vi "getSerializedData.vi"(0 "reference":refnum<class "PackageNode.lvclass">, 5 "error in (no error)":errorcluster) -> (14 "reference out":refnum<class "PackageNode.lvclass">, 15 "parent":refnum<class "AbstractNode.lvclass">, 16 "children":refnum<class "AbstractNode.lvclass">[](array[class]), 17 "xmlOut":string, 19 "error out":errorcluster)   [LabVIEW 2014, in "PackageNode.lvclass"]
doc: "getSerializedData"
uses:
  <resource>/Framework/Providers/Open_GDS/UML/PackageNode_class/PackageNode.lvclass
  <resource>/Framework/Providers/Open_GDS/UML/AbstractNode_class/AbstractNode.lvclass
  <resource>/Framework/Providers/Open_GDS/UML/AbstractNode_class/ObjectReference.ctl
  <resource>/Framework/Providers/Open_GDS/UML/General/Rectangle/Rectangle Rectangle2D.ctl
  <resource>/Framework/Providers/Open_GDS/UML/MultiLineString_class/ObjectReference.ctl
  <resource>/Framework/Providers/Open_GDS/UML/MultiLineString_class/MultiLineString.lvclass
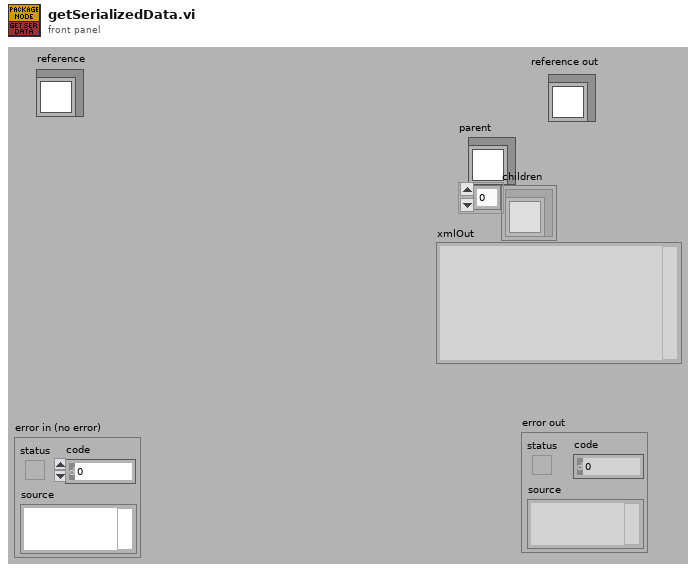
[diagram p1: front panel]
types:
  T1 = typedef "AbstractNode.lvclass/ObjectReference.ctl" = refnum<k1>
  T2 = typedef "Rectangle Rectangle2D.ctl" = cluster{"x":dbl, "y":dbl, "width":dbl, "height":dbl}
  T3 = typedef "MultiLineString.lvclass/ObjectReference.ctl" = refnum<k1>
  T4 = cluster{"Base class":cluster{"Base class":cluster{"parent":T1, "children":T1[], "Hidden":bool}, "bounds":T2}, "name":string, "contents":T3, "DEFAULT_TOP_WIDTH":i32, "DEFAULT_TOP_HEIGHT":i32, "DEFAULT_WIDTH":i32, "DEFAULT_HEIGHT":i32, "NAME_GAP":i32, "XGAP":i32, "YGAP":i32, "Collapsed":bool, "Note color":u32, "Justification":u16}
  T5 = typedef "PackageNode.lvclass/ObjectAttributes.ctl" = cluster{"Base class":T6, "name":string, "contents":refnum<class "MultiLineString.lvclass">, "DEFAULT_TOP_WIDTH":i32, "DEFAULT_TOP_HEIGHT":i32, "DEFAULT_WIDTH":i32, "DEFAULT_HEIGHT":i32, "NAME_GAP":i32, "XGAP":i32, "YGAP":i32, "Collapsed":bool, "Note color":u32, "Justification":u16}
  T6 = typedef "RectangularNode.lvclass/ObjectAttributes.ctl" = cluster{"Base class":T7, "bounds":T2}
  T7 = typedef "AbstractNode.lvclass/ObjectAttributes.ctl" = cluster{"parent":refnum<class "AbstractNode.lvclass">, "children":refnum<class "AbstractNode.lvclass">[], "Hidden":bool}
  T8 = cluster{"Attributes":cluster{"Base class":cluster{"Base class":cluster{"parent":T1, "children":T1[], "Hidden":bool}, "bounds":T2}, "name":string, "contents":T3, "DEFAULT_TOP_WIDTH":i32, "DEFAULT_TOP_HEIGHT":i32, "DEFAULT_WIDTH":i32, "DEFAULT_HEIGHT":i32, "NAME_GAP":i32, "XGAP":i32, "YGAP":i32, "Collapsed":bool, "Note color":u32, "Justification":u16}, "text":string}
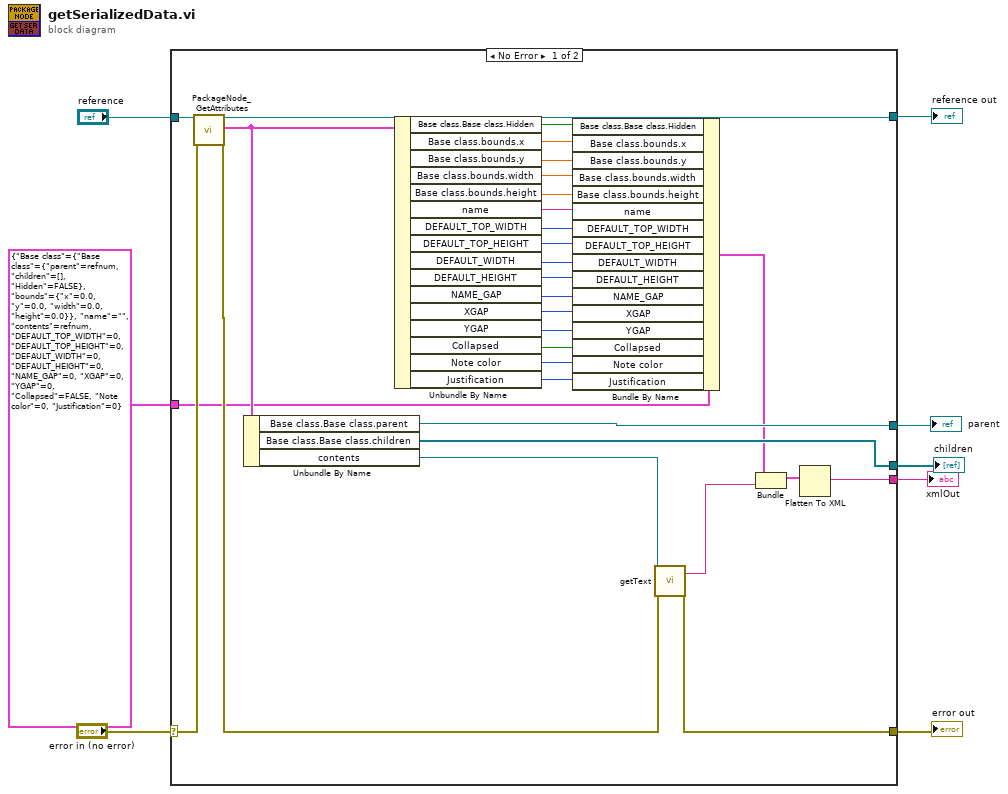
[diagram p0: block diagram]
diagram:
  n1 = case shown="No Error" "error in (no error)" {
    selector: "error in (no error)" -> [w38 w39]
    tunnel: "reference" -> [w37 w40]
    tunnel: [w31 w39] -> w6
    tunnel: [w36 w40] -> w5
    tunnel: [w30 _] -> w4
    tunnel: [w29 _] -> w3
    tunnel: [w28 _] -> w2
    tunnel: T4 {"Base class"={"Base class"={"parent"=refnum, "children"=[], "Hidden"=FALSE}, "bounds"={"x"=0.0, "y"=0.0, "width"=0.0, "height"=0.0}}, "name"="", "contents"=refnum, "DEFAULT_TOP_WIDTH"=0, "DEFAULT_TOP_HEIGHT"=0, "DEFAULT_WIDTH"=0, "DEFAULT_HEIGHT"=0, "NAME_GAP"=0, "XGAP"=0, "YGAP"=0, "Collapsed"=FALSE, "Note color"=0, "Justification"=0} ("Attributes") -> [w19 _]
    frame No Error {
      n2 = call <resource>:"PackageNode_GetAttributes.vi"("reference in"=w37, "error in (no error)"=w38) -> ("reference out"=w36:refnum<class "PackageNode.lvclass">, "Attributes"=w21:T5, "error out"=w32:errorcluster)  [unwired: 15 out]
      n3 = Unbundle By Name(w21) -> ("Base class.Base class.parent"=w30:refnum<class "AbstractNode.lvclass">, "Base class.Base class.children"=w29:refnum<class "AbstractNode.lvclass">[], "contents"=w33:refnum<class "MultiLineString.lvclass">)
      n4 = Unbundle By Name(w21) -> ("Base class.Base class.Hidden"=w11:bool, "Base class.bounds.x"=w18:dbl, "Base class.bounds.y"=w17:dbl, "Base class.bounds.width"=w16:dbl, "Base class.bounds.height"=w27:dbl, "name"=w26:string, "DEFAULT_TOP_WIDTH"=w25:i32, "DEFAULT_TOP_HEIGHT"=w24:i32, "DEFAULT_WIDTH"=w23:i32, "DEFAULT_HEIGHT"=w22:i32, "NAME_GAP"=w15:i32, "XGAP"=w14:i32, "YGAP"=w13:i32, "Collapsed"=w12:bool, "Note color"=w10:u32, "Justification"=w9:u16)
      n5 = Bundle By Name(cluster=w19, "Base class.Base class.Hidden"=w11, "Base class.bounds.x"=w18, "Base class.bounds.y"=w17, "Base class.bounds.width"=w16, "Base class.bounds.height"=w27, "name"=w26, "DEFAULT_TOP_WIDTH"=w25, "DEFAULT_TOP_HEIGHT"=w24, "DEFAULT_WIDTH"=w23, "DEFAULT_HEIGHT"=w22, "NAME_GAP"=w15, "XGAP"=w14, "YGAP"=w13, "Collapsed"=w12, "Note color"=w10, "Justification"=w9) -> (w20:T4)
      n6 = call-dynamic "getText.vi"("reference"=w33, "error in (no error)"=w32) -> ("text"=w34:string, "error out"=w31:errorcluster)  [unwired: 16 out]
      n7 = Bundle("Attributes"=w20, "text"=w34) -> (w35:T8)  [unwired: 1 out]
      n8 = Flatten To XML(anything=w35) -> (xml string=w28:string)
    }
    frame Error {
    }
  }
  "reference out" <- w5
  "error out" <- w6
  "parent" <- w4
  "children" <- w3
  "xmlOut" <- w2
